vi "workbook set custom property datetime.vi"(8 "error in (no error)":errorcluster, 9 "datetime":T1, 10 "name":string, 11 "workbook":u32) -> (0 "error out":errorcluster, 1 "datetime out":T1, 3 "function return":u32(ring))   [LabVIEW 8.6]
doc: "lxw_error workbook_set_custom_property_datetime(lxw_workbook workbook, const char *name, lxw_datetime *datetime);"
uses:
  pending_lvxlsxwriter/xlsxwriter.dll
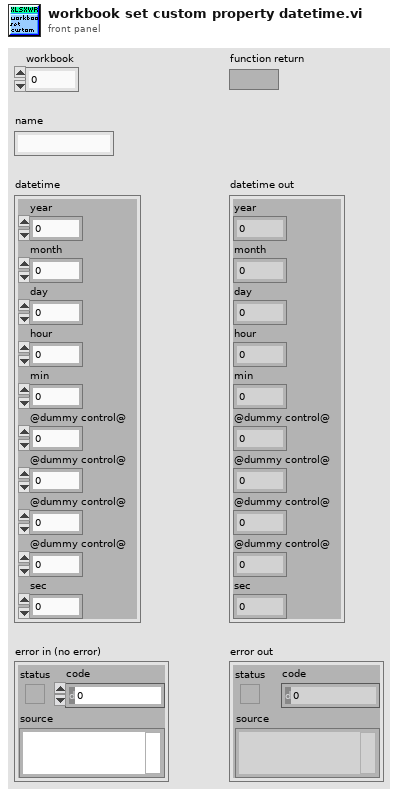
[diagram p1: front panel]
types:
  T1 = cluster{"year":i32, "month":i32, "day":i32, "hour":i32, "min":i32, "@dummy control@":i8, "@dummy control@":i8, "@dummy control@":i8, "@dummy control@":i8, "sec":dbl}
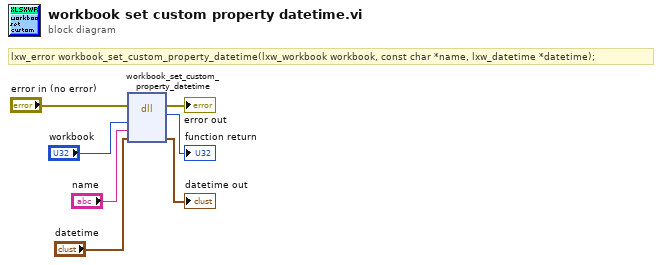
[diagram p0: block diagram]
diagram:
  # "lxw_error workbook_set_custom_property_datetime(lxw_workbook workbook, const char *name, lxw_datetime *datetime);"
  n1 = dll-call lib="C:/Users/WDAGUtilityAccount/Desktop/pending_lvxlsxwriter/xlsxwriter.*" fn="workbook_set_custom_property_datetime"(error in="error in (no error)", "workbook"="workbook", "name"="name", "datetime"="datetime") -> (error out=→"error out":errorcluster, →"function return":u32, "datetime"=→"datetime out":T1)  [unwired: 4 in, 1 out]
